vi "ReadControl.vi"(2 "reference":refnum<vi>) -> (1 "Control":T6)   [LabVIEW 2013]
uses:
  <vilib>/Utility/miscctls.llb/LVBoundsTypeDef.ctl
  <vilib>/Utility/miscctls.llb/LVRectTypeDef.ctl
  <vilib>/Utility/miscctls.llb/LVPositionTypeDef.ctl
  <vilib>/Utility/miscctls.llb/LVDataSocketStatusTypeDef.ctl
  <vilib>/Utility/miscctls.llb/LVKeyNavTypeDef.ctl
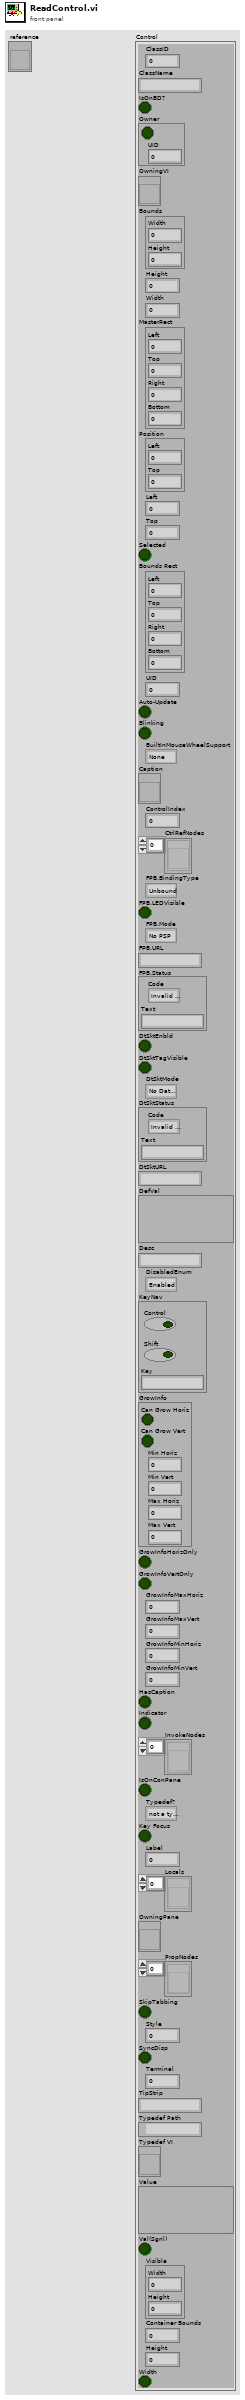
[diagram p1: front panel]
types:
  T1 = typedef "LVBoundsTypeDef.ctl" = cluster{"Width":u32, "Height":u32}
  T2 = typedef "LVRectTypeDef.ctl" = cluster{"Left":i16, "Top":i16, "Right":i16, "Bottom":i16}
  T3 = typedef "LVPositionTypeDef.ctl" = cluster{"Left":i32, "Top":i32}
  T4 = typedef "LVDataSocketStatusTypeDef.ctl" = cluster{"Code":enum32{"Invalid Status", "Unconnected", "Active", "Idle", "Error", "Connecting"}, "Text":string}
  T5 = typedef "LVKeyNavTypeDef.ctl" = cluster{"Control":bool, "Shift":bool, "Key":string}
  T6 = cluster{"ClassID":u32, "ClassName":string, "IsOnBD?":bool, "Owner":cluster{bool, "UID":i32}, "OwningVI":refnum<vi>, "Bounds":T1, "Height":u32, "Width":u32, "MasterRect":T2, "Position":T3, "Left":i32, "Top":i32, "Selected":bool, "Bounds Rect":T2, "UID":i32, "Auto-Update":bool, "Blinking":bool, "BuiltInMouseWheelSupport":enum16{"None", "On Hover", "On Key Focus", "On Hover or Key Focus"}, "Caption":refnum<vi>, "ControlIndex":i32, "CtrlRefNodes":refnum<vi>[], "FPB.BindingType":enum32{"Unbound", "Bound To PSP URL", "Bound To Variable Shortcut"}, "FPB.LEDVisible":bool, "FPB.Mode":enum32{"No PSP", "Read", "Write", "Write & Read"}, "FPB.URL":string, "FPB.Status":T4, "DtSktEnbld":bool, "DtSktTagVisible":bool, "DtSktMode":enum32{"No DataSocket", "Publish", "Subscribe", "Publish & Subscribe"}, "DtSktStatus":T4, "DtSktURL":string, "DefVal":variant, "Desc":string, "DisabledEnum":enum8{"Enabled", "Disabled", "Disabled and Grayed Out"}, "KeyNav":T5, "GrowInfo":cluster{"Can Grow Horiz":bool, "Can Grow Vert":bool, "Min Horiz":i16, "Min Vert":i16, "Max Horiz":i16, "Max Vert":i16}, "GrowInfoHorizOnly":bool, "GrowInfoVertOnly":bool, "GrowInfoMaxHoriz":i16, "GrowInfoMaxVert":i16, "GrowInfoMinHoriz":i16, "GrowInfoMinVert":i16, "HasCaption":bool, "Indicator":bool, "InvokeNodes":refnum<vi>[], "IsOnConPane":bool, "Typedef?":enum32{"not a typedef", "typedef", "strict typedef", "class private data"}, "Key Focus":bool, "Label":i32, "Locals":refnum<vi>[], "OwningPane":refnum<vi>, "PropNodes":refnum<vi>[], "SkipTabbing":bool, "Style":u32, "SyncDisp":bool, "Terminal":i32, "TipStrip":string, "Typedef Path":path, "Typedef VI":refnum<vi>, "Value":variant, "Val(Sgnl)":bool, "Visible":T1, "Container Bounds":u32, "Height":u32, "Width":bool}
  T7 = enum16{"None", "On Hover", "On Key Focus", "On Hover or Key Focus"}
  T8 = enum32{"Unbound", "Bound To PSP URL", "Bound To Variable Shortcut"}
  T9 = enum32{"No PSP", "Read", "Write", "Write & Read"}
  T10 = enum32{"No DataSocket", "Publish", "Subscribe", "Publish & Subscribe"}
  T11 = enum8{"Enabled", "Disabled", "Disabled and Grayed Out"}
  T12 = cluster{"Can Grow Horiz":bool, "Can Grow Vert":bool, "Min Horiz":i16, "Min Vert":i16, "Max Horiz":i16, "Max Vert":i16}
  T13 = enum32{"not a typedef", "typedef", "strict typedef", "class private data"}
  T14 = cluster{"ClassID":u32, "ClassName":string, "IsOnBD?":bool, "Cluster":cluster{bool, "UID":i32}, "OwningVI":refnum<vi>, "Bounds":T1, "Height":u32, "Width":u32, "MasterRect":T2, "Position":T3, "Left":i32, "Top":i32, "Selected":bool, "Bounds Rect":T2, "UID":i32, "Auto-Update":bool, "Blinking":bool, "BuiltInMouseWheelSupport":enum16{"None", "On Hover", "On Key Focus", "On Hover or Key Focus"}, "Caption":refnum<vi>, "ControlIndex":i32, "CtrlRefNodes":refnum<vi>[], "FPB.BindingType":enum32{"Unbound", "Bound To PSP URL", "Bound To Variable Shortcut"}, "FPB.LEDVisible":bool, "FPB.Mode":enum32{"No PSP", "Read", "Write", "Write & Read"}, "FPB.URL":string, "FPB.Status":T4, "DtSktEnbld":bool, "DtSktTagVisible":bool, "DtSktMode":enum32{"No DataSocket", "Publish", "Subscribe", "Publish & Subscribe"}, "DtSktStatus":T4, "DtSktURL":string, "DefVal":variant, "Desc":string, "DisabledEnum":enum8{"Enabled", "Disabled", "Disabled and Grayed Out"}, "KeyNav":T5, "GrowInfo":cluster{"Can Grow Horiz":bool, "Can Grow Vert":bool, "Min Horiz":i16, "Min Vert":i16, "Max Horiz":i16, "Max Vert":i16}, "GrowInfoHorizOnly":bool, "GrowInfoVertOnly":bool, "GrowInfoMaxHoriz":i16, "GrowInfoMaxVert":i16, "GrowInfoMinHoriz":i16, "GrowInfoMinVert":i16, "HasCaption":bool, "Indicator":bool, "InvokeNodes":refnum<vi>[], "IsOnConPane":bool, "Typedef?":enum32{"not a typedef", "typedef", "strict typedef", "class private data"}, "Key Focus":bool, "UID":i32, "Locals":refnum<vi>[], "OwningPane":refnum<vi>, "PropNodes":refnum<vi>[], "SkipTabbing":bool, "Style":u32, "SyncDisp":bool, "UID":i32, "TipStrip":string, "Typedef Path":path, "Typedef VI":refnum<vi>, "Value":variant, "Visible":bool, "Container Bounds":T1, "Height":u32, "Width":u32, "Is XControl?":bool}
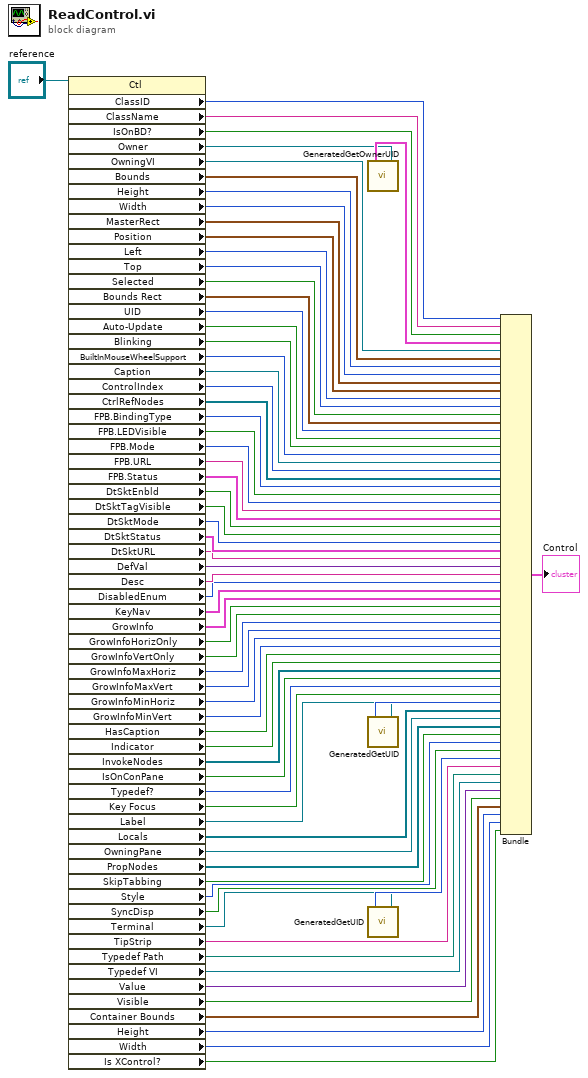
[diagram p0: block diagram]
diagram:
  n1 = property class="Ctl"(reference="reference") -> ("ClassID"=w69:u32, "ClassName"=w68:string, "IsOnBD?"=w67:bool, "Owner"=w65:refnum<vi>, "OwningVI"=w64:refnum<vi>, "Bounds"=w63:T1, "Height"=w62:u32, "Width"=w61:u32, "MasterRect"=w60:T2, "Position"=w59:T3, "Left"=w58:i32, "Top"=w57:i32, "Selected"=w56:bool, "Bounds Rect"=w55:T2, "UID"=w54:i32, "Auto-Update"=w53:bool, "Blinking"=w52:bool, "BuiltInMouseWheelSupport"=w51:T7, "Caption"=w50:refnum<vi>, "ControlIndex"=w49:i32, "CtrlRefNodes"=w48:refnum<vi>[], "FPB.BindingType"=w47:T8, "FPB.LEDVisible"=w46:bool, "FPB.Mode"=w45:T9, "FPB.URL"=w44:string, "FPB.Status"=w43:T4, "DtSktEnbld"=w42:bool, "DtSktTagVisible"=w41:bool, "DtSktMode"=w40:T10, "DtSktStatus"=w39:T4, "DtSktURL"=w38:string, "DefVal"=w37:variant, "Desc"=w36:string, "DisabledEnum"=w35:T11, "KeyNav"=w34:T5, "GrowInfo"=w33:T12, "GrowInfoHorizOnly"=w32:bool, "GrowInfoVertOnly"=w31:bool, "GrowInfoMaxHoriz"=w30:i16, "GrowInfoMaxVert"=w29:i16, "GrowInfoMinHoriz"=w28:i16, "GrowInfoMinVert"=w27:i16, "HasCaption"=w26:bool, "Indicator"=w25:bool, "InvokeNodes"=w24:refnum<vi>[], "IsOnConPane"=w23:bool, "Typedef?"=w22:T13, "Key Focus"=w21:bool, "Label"=w19:refnum<vi>, "Locals"=w18:refnum<vi>[], "OwningPane"=w17:refnum<vi>, "PropNodes"=w16:refnum<vi>[], "SkipTabbing"=w15:bool, "Style"=w14:u32, "SyncDisp"=w13:bool, "Terminal"=w11:refnum<vi>, "TipStrip"=w10:string, "Typedef Path"=w9:path, "Typedef VI"=w8:refnum<vi>, "Value"=w7:variant, "Visible"=w6:bool, "Container Bounds"=w5:T1, "Height"=w4:u32, "Width"=w3:u32, "Is XControl?"=w2:bool)  [unwired: 1 in, 2 out]
  n2 = call "GeneratedGetOwnerUID.vi"("Generic in"=w65) -> ("Cluster"=w66:cluster{bool, "UID":i32})
  n3 = call "GeneratedGetUID.vi"("Text in"=w19) -> ("UID"=w20:i32)
  n4 = call "GeneratedGetUID.vi"("Text in"=w11) -> ("UID"=w12:i32)
  n5 = Bundle("ClassID"=w69, "ClassName"=w68, "IsOnBD?"=w67, "Cluster"=w66, "OwningVI"=w64, "Bounds"=w63, "Height"=w62, "Width"=w61, "MasterRect"=w60, "Position"=w59, "Left"=w58, "Top"=w57, "Selected"=w56, "Bounds Rect"=w55, "UID"=w54, "Auto-Update"=w53, "Blinking"=w52, "BuiltInMouseWheelSupport"=w51, "Caption"=w50, "ControlIndex"=w49, "CtrlRefNodes"=w48, "FPB.BindingType"=w47, "FPB.LEDVisible"=w46, "FPB.Mode"=w45, "FPB.URL"=w44, "FPB.Status"=w43, "DtSktEnbld"=w42, "DtSktTagVisible"=w41, "DtSktMode"=w40, "DtSktStatus"=w39, "DtSktURL"=w38, "DefVal"=w37, "Desc"=w36, "DisabledEnum"=w35, "KeyNav"=w34, "GrowInfo"=w33, "GrowInfoHorizOnly"=w32, "GrowInfoVertOnly"=w31, "GrowInfoMaxHoriz"=w30, "GrowInfoMaxVert"=w29, "GrowInfoMinHoriz"=w28, "GrowInfoMinVert"=w27, "HasCaption"=w26, "Indicator"=w25, "InvokeNodes"=w24, "IsOnConPane"=w23, "Typedef?"=w22, "Key Focus"=w21, "UID"=w20, "Locals"=w18, "OwningPane"=w17, "PropNodes"=w16, "SkipTabbing"=w15, "Style"=w14, "SyncDisp"=w13, "UID"=w12, "TipStrip"=w10, "Typedef Path"=w9, "Typedef VI"=w8, "Value"=w7, "Visible"=w6, "Container Bounds"=w5, "Height"=w4, "Width"=w3, "Is XControl?"=w2) -> (→"Control":T14)  [unwired: 1 in]
